vi "Write MMF Header (SubVI).vi"(0 "FILE REF IN":refnum<file>, 8 "Base Name":string="Rawdata", 10 "Output File Path":path=path "D:/Rawdata") -> (14 "FILE REF OUT":refnum<file>)   [LabVIEW 2015]
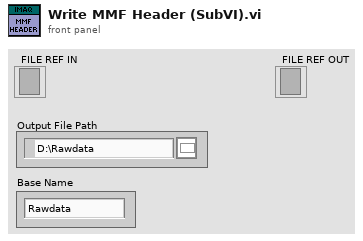
[diagram p1: front panel]
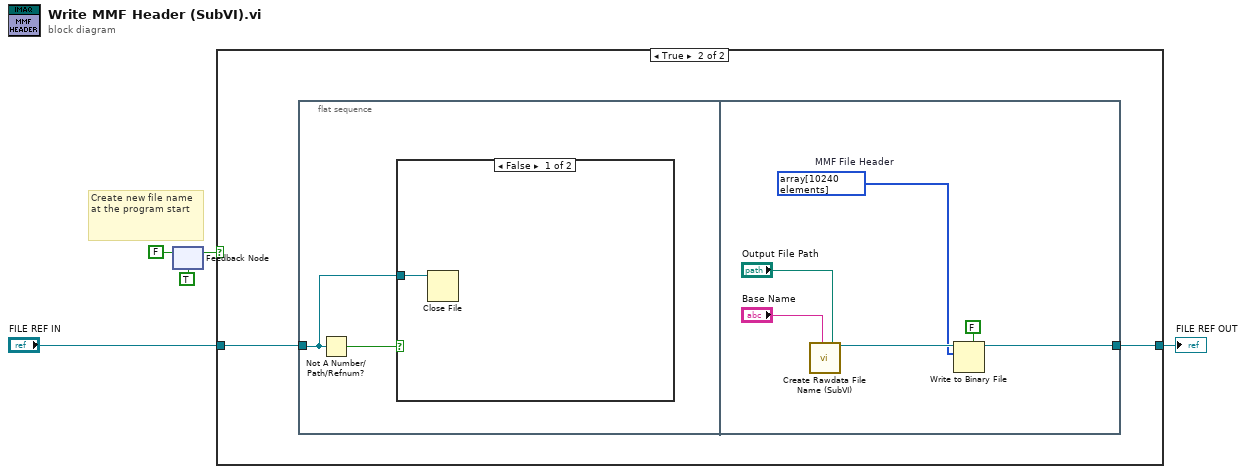
[diagram p0: block diagram]
diagram:
  # "Create new file name at the program start"
  n1 = feedback #1(TRUE) -> (w2:bool)
  n2 = feedback-in #1(FALSE) -> ()
  n3 = case shown="True" w2 {
    tunnel: "FILE REF IN" -> [w6 w8]
    tunnel: [w6 w7] -> w4
    frame False {
    }
    frame True {
      n4 = flat-sequence {
        tunnel: w8 -> [w9]
        tunnel: [w14] -> w7
        frame #0 {
          n5 = Not A Number/Path/Refnum?(number/path/refnum=w9) -> (NaN/Path/Refnum?=w10:bool)
          n6 = case shown="False" w10 {
            tunnel: w9 -> [w11 _]
            frame False {
              n7 = Close File(refnum=w11) -> ()  [unwired: 1 in, 2 out]
            }
            frame True {
            }
          }
        }
        frame #1 {
          w13 = u8[] array[10240 elements]  # MMF File Header
          n8 = call "Create Rawdata File Name (SubVI).vi"("Base Name"="Base Name", "Output File Path"="Output File Path") -> ("Byte Stream File out"=w17:refnum<file>)  [unwired: 17 in]
          n9 = Write to Binary File(file (use dialog)=w17, data=w13, 5:FALSE ("prepend array or string size? (T)")) -> (refnum out=w14:refnum<file>)  [unwired: 3 in, 2 out]
        }
      }
    }
  }
  "FILE REF OUT" <- w4
